vi "EPS-Query Operation Value.vi"(8 "error in":errorcluster, 10 "Value Type":T1, 11 "EPS Setting In":T2) -> (0 "error out":errorcluster, 2 "Value":dbl, 3 "EPS Setting Out":T2)   [LabVIEW 2018]
uses:
  Data Def/EPS-Setting.ctl
  Data Def/EPS-Value Type.ctl
  Data Def/EPS-Access Mode.ctl
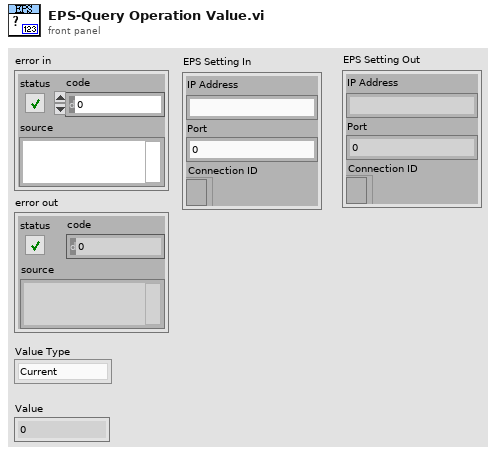
[diagram p1: front panel]
types:
  T1 = typedef "EPS-Value Type.ctl" = enum16{"Current", "Vlotage", "Power"}
  T2 = typedef "EPS-Setting.ctl" = cluster{"IP Address":string, "Port":u16, "Connection ID":refnum<k5>}
  T3 = typedef "EPS-Access Mode.ctl" = enum16{"Read", "Write"}
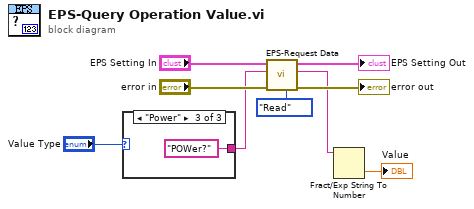
[diagram p0: block diagram]
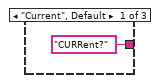
[diagram p2: hidden frame]
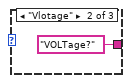
[diagram p3: hidden frame]
diagram:
  n1 = case shown="\"Power\"" "Value Type" {
    tunnel: ["CURRent?" ("Requst Data") "VOLTage?" ("Requst Data") "POWer?" ("Requst Data")] -> w6
    frame "Current", Default {
    }
    frame "Vlotage" {
    }
    frame "Power" {
    }
  }
  n2 = call "EPS-Request Data.vi"("Access Mode"=EPS-Access_Mode."Read", "error in"="error in", "Requst Data"=w6, "EPS Setting In"="EPS Setting In") -> ("error out"=→"error out":errorcluster, "Response Data"=w2:string, "EPS Setting Out"=→"EPS Setting Out":T2)  [unwired: 5 in]
  n3 = Fract/Exp String To Number(string=w2) -> (number=→"Value":dbl)  [unwired: 3 in, 1 out]
